vi "VeristandStop.vi"(8 "error in (no error)":errorcluster, 10 "CloseApp?":bool, 11 "Project Ref in":T1) -> (0 "error out":errorcluster)   [LabVIEW 2015, in "MiscHelperVIs.lvlib"]
uses:
  MiscHelperVIs.lvlib
  <vilib>/NI Veristand/Execution/Project/Project Ref.ctl
  NationalInstruments.VeriStand.ClientAPI
  <vilib>/NI Veristand/Execution/Project/NI_VS Project ExecutionAPI.lvlib
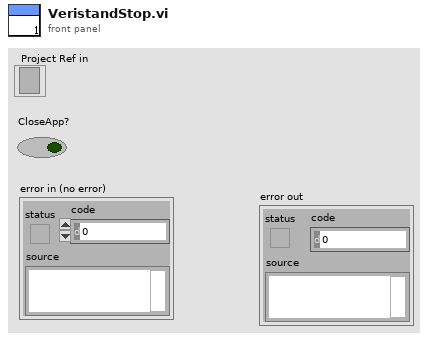
[diagram p1: front panel]
types:
  T1 = typedef "NI_VS Project ExecutionAPI.lvlib/Project Ref.ctl" = refnum<k24>
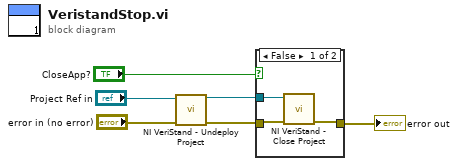
[diagram p0: block diagram]
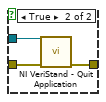
[diagram p2: hidden frame]
diagram:
  n1 = call <vilib>:"NI VeriStand - Undeploy Project.vi"("error in (no error)"="error in (no error)", "Project Ref in"="Project Ref in") -> ("error out"=w2:errorcluster, "Project Ref out"=w1:T1)  [unwired: 8 in]
  n2 = case shown="False" "CloseApp?" {
    tunnel: w1 -> [w9 w12]
    tunnel: w2 -> [w8 w11]
    tunnel: [w7 w10] -> w3
    frame False {
      n3 = call <vilib>:"NI VeriStand - Close Project.vi"("error in (no error)"=w8, "Project Ref in"=w9) -> ("error out"=w7:errorcluster)  [unwired: 8 in, 1 out]
    }
    frame True {
      n4 = call <vilib>:"NI VeriStand - Quit Application.vi"("error in (no error)"=w11, "Project Ref in"=w12) -> ("error out"=w10:errorcluster)  [unwired: 8 in, 1 out]
    }
  }
  "error out" <- w3
